vi "Format JSON String.vi"(10 "String":string) -> (2 "Formatted Basic String":string)   [LabVIEW 2015, in "JSON.lvlib"]
uses:
  JSON.lvlib
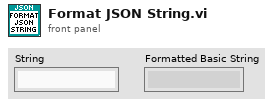
[diagram p1: front panel]
types:
  T1 = cluster{"replace string (\"\")":string, "replace string (\"\") 2":string}[]
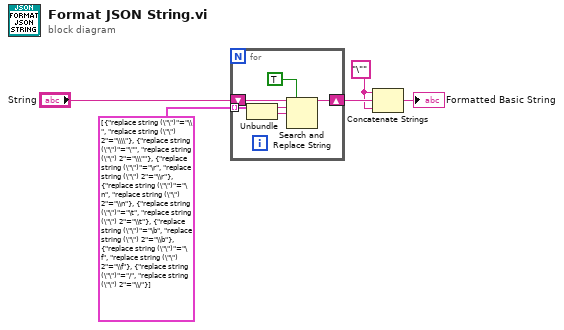
[diagram p0: block diagram]
diagram:
  w2 = "\"" ("string")
  n1 = for {
    tunnel: T1 [{"replace string (\"\")"="\\", "replace string (\"\") 2"="\\\\"}, {"replace string (\"\")"="\"", "replace string (\"\") 2"="\\\""}, {"replace string (\"\")"="\r", "replace string (\"\") 2"="\\r"}, {"replace string (\"\")"="\n", "replace string (\"\") 2"="\\n"}, {"replace string (\"\")"="\t", "replace string (\"\") 2"="\\t"}, {"replace string (\"\")"="\b", "replace string (\"\") 2"="\\b"}, {"replace string (\"\")"="\f", "replace string (\"\") 2"="\\f"}, {"replace string (\"\")"="/", "replace string (\"\") 2"="\\/"}] -> [w9] mode=indexing
    shift-right: [w6] -> w3
    shift-left: "String" -> [w11]
    n2 = Unbundle(w9) -> ("replace string (\"\")"=w8:string, "replace string (\"\") 2"=w7:string)
    n3 = Search and Replace String(replace all?=TRUE ("replace all? (F)"), input string=w11, search string=w8, replace string=w7) -> (result string=w6:string)  [unwired: 4 in, 3 out]
  }
  n4 = Concatenate Strings(w2, w3, w2) -> (→"Formatted Basic String":string)
